vi "Base Init.vi"(9 "Actor":refnum<class "Actor.lvclass">, 10 "Alias":string) -> (0 "Reported Is Normal":bool, 1 "Reported":bool, 2 "Actor":refnum<class "Actor.lvclass">, 4 "Reported Error":errorcluster)   [LabVIEW 2020, in "jettl.lvlib" / "Actor.lvlib"]
uses:
  Actor.lvlib
  Actor/Actor.lvclass
  Attributes.ctl
  Msg/Msg.lvclass
  Implemented Msgs.ctl
  Base Actor/Base Actor.lvclass
  C:/git/jettl/src/jettl/jettl/Actor/Actor/Actor.lvclass
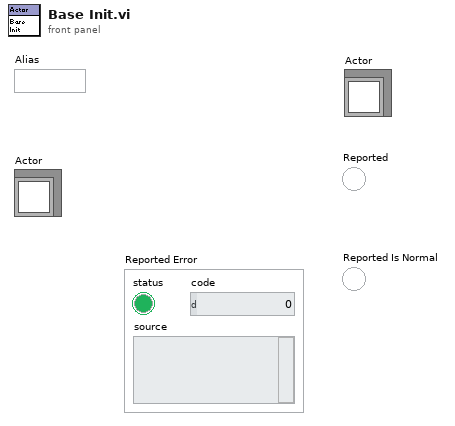
[diagram p1: front panel]
types:
  T1 = typedef "jettl.lvlib/Actor.lvlib/Attributes.ctl" = cluster{"Alias":string, "Address":refnum<user-event>, "Register":refnum<event-registration>, "Implemented Msgs":T2, "Path":path}
  T2 = typedef "jettl.lvlib/Actor.lvlib/Implemented Msgs.ctl" = set{refnum<class "Msg.lvclass">}
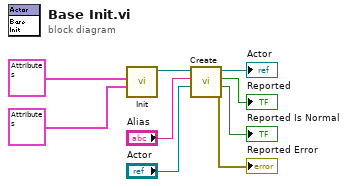
[diagram p0: block diagram]
diagram:
  n1 = call "Init.vi"("Creator Attributes"=T1 {"Alias"="", "Address"=refnum, "Register"=refnum, "Implemented Msgs"={}, "Path"=path ""}, "Self Attributes"=T1 {"Alias"="", "Address"=refnum, "Register"=refnum, "Implemented Msgs"={}, "Path"=path ""}) -> ("Base Actor out"=w7:refnum<class "Base Actor.lvclass">)  [unwired: 9 in]
  n2 = call-dynamic "Create.vi"("Actor"="Actor", "Alias"="Alias", "Base Actor in"=w7) -> ("Reported Error"=→"Reported Error":errorcluster, "Reported Is Normal"=→"Reported Is Normal":bool, "Reported"=→"Reported":bool, "Base Actor out"=→"Actor":refnum<class "Base Actor.lvclass">)  [unwired: 5 in]
